vi "API_GetSysemMetrics.vi"(8 "error in (no error)":errorcluster caption="错误输入（无错误）", 11 "Index":T1) -> (0 "error out":errorcluster caption="错误输出", 3 "Para":i32)   [LabVIEW 2012, in "API.lvlib"]
uses:
  API.lvlib
  SM.ctl
  user32.dll
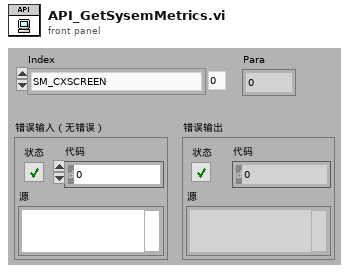
[diagram p1: front panel]
types:
  T1 = typedef "SM.ctl" = enum16{"SM_CXSCREEN", "SM_CYSCREEN", "SM_CXVSCROLL", "SM_CYHSCROLL", "SM_CYCAPTION", "SM_CXBORDER;", "SM_CYBORDER", "SM_CXDLGFRAME", "SM_CYDLGFRAME", "SM_CYVTHUMB", "SM_CXHTHUMB", "SM_CXICON", "SM_CYICON", "SM_CXCURSOR", "SM_CYCURSOR", "SM_CYMENU", "SM_CXFULLSCREEN", "SM_CYFULLSCREEN", "SM_CYKANJIWINDOW", "SM_MOUSEPRESENT", "SM_CYVSCROLL", "SM_CXHSCROLL", "SM_DEBUG", "SM_SWAPBUTTON", "SM_RESERVED1", "SM_RESERVED2", "SM_RESERVED3", "SM_RESERVED4", "SM_CXMIN", "SM_CYMIN", "SM_CXSIZE", "SM_CYSIZE", "SM_CXFRAME", "SM_CYFRAME", "SM_CXMINTRACK", "SM_CYMINTRACK", "SM_CXDOUBLECLK", "SM_CYDOUBLECLK", "SM_CXICONSPACING", "SM_CYICONSPACING", "SM_MENUDROPALIGNMENT", "SM_PENWINDOWS", "SM_DBCSENABLED", "SM_CMOUSEBUTTONS", "SM_SECURE", "SM_CXEDGE", "SM_CYEDGE", "SM_CXMINSPACING", "SM_CYMINSPACING", "SM_CXSMICON", "SM_CYSMICON", "SM_CYSMCAPTION", "SM_CXSMSIZE", "SM_CYSMSIZE", "SM_CXMENUSIZE", "SM_CYMENUSIZE", "SM_ARRANGE", "SM_CXMINIMIZED", "SM_CYMINIMIZED", "SM_CXMAXTRACK", "SM_CYMAXTRACK", "SM_CXMAXIMIZED", "SM_CYMAXIMIZED", "SM_NETWORK", "Not Defined 1", "Not Defined 2", "Not Defined 3", "SM_CLEANBOOT", "SM_CXDRAG", "SM_CYDRAG", "SM_SHOWSOUNDS", "SM_CXMENUCHECK", "SM_CYMENUCHECK", "SM_SLOWMACHINE", "SM_MIDEASTENABLED", "SM_MOUSEWHEELPRESENT ", "SM_XVIRTUALSCREEN", "SM_YVIRTUALSCREEN", "SM_CXVIRTUALSCREEN", "SM_CYVIRTUALSCREEN", "SM_CMONITORS", "SM_SAMEDISPLAYFORMAT", "SM_IMMENABLED", "SM_CXFOCUSBORDER", "SM_CYFOCUSBORDER"}
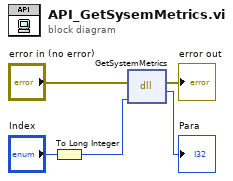
[diagram p0: block diagram]
diagram:
  n1 = To Long Integer(number="Index") -> (32bit integer=w4:i32)
  n2 = dll-call lib="USER32.DLL" fn="GetSystemMetrics"(error in="error in (no error)", "Index"=w4) -> (error out=→"error out":errorcluster, "返回类型"=→"Para":i32)  [unwired: 3 in, 1 out]
